vi "jettl Msg Last Ack Queue.vi"(10 "Queue":refnum<class "Queue.lvclass">) -> (2 "Msg Strategy":refnum<class "Msg Strategy.lvclass">)   [LabVIEW 2021, in "jettl.lvlib" / "jettl Msg Last Ack Queue.lvlib"]
uses:
  jettl Msg Last Ack Queue.lvlib
  Queue/Queue.lvclass
  Msg Strategy/Msg Strategy.lvclass
  Last Ack Queue Msg Strategy/Last Ack Queue Msg Strategy.lvclass
  C:/git/jettl/src/jettl/Msg Strategy/Msg Strategy.lvclass
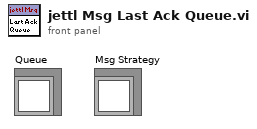
[diagram p1: front panel]
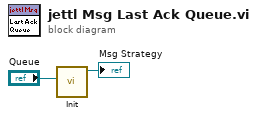
[diagram p0: block diagram]
diagram:
  n1 = call "Init.vi"("Queue"="Queue") -> ("Last Ack Queue Msg Strategy out"=→"Msg Strategy":refnum<class "Last Ack Queue Msg Strategy.lvclass">)  [unwired: 10 in]
